vi "QueryServer_SetAnalogInputData.vi"(6 "error in (no error)":errorcluster, 8 "AnalogInputData":T1, 9 "gRPCid":T2) -> (0 "error out":errorcluster, 3 "gRPCid out":T2)   [LabVIEW 2019, in "labview-grpc-query-server.lvlib"]
uses:
  labview-grpc-query-server.lvlib
  VIs/grpcId.ctl
  QueryServer_AnalogInputData.ctl
  d149c175-cf88-4dc1-b2b5-9725cea78de2.vi
  VIs/gprc-support.lvlib
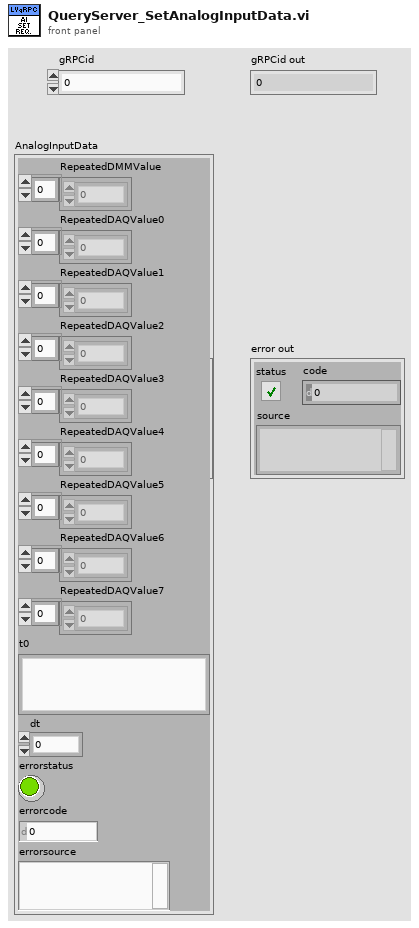
[diagram p1: front panel]
types:
  T1 = typedef "labview-grpc-query-server.lvlib/QueryServer_AnalogInputData.ctl" = cluster{"RepeatedDMMValue":sgl[], "RepeatedDAQValue0":sgl[], "RepeatedDAQValue1":sgl[], "RepeatedDAQValue2":sgl[], "RepeatedDAQValue3":sgl[], "RepeatedDAQValue4":sgl[], "RepeatedDAQValue5":sgl[], "RepeatedDAQValue6":sgl[], "RepeatedDAQValue7":sgl[], "t0":string, "dt":sgl, "errorstatus":bool, "errorcode":i32, "errorsource":string}
  T2 = typedef "gprc-support.lvlib/grpcId.ctl" = u64
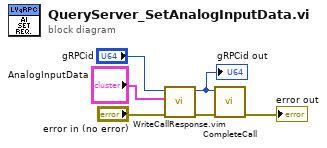
[diagram p0: block diagram]
diagram:
  n1 = call "WriteCallResponse.vim"("error in (no error)"="error in (no error)", "Response Data"="AnalogInputData", "gRPCid in"="gRPCid") -> ("error out"=w5:errorcluster, "gRPCid"=w3:T2)  [unwired: 7 in]
  "gRPCid out" <- w3
  n2 = call "CompleteCall.vi"("gRPCid"=w3, "error in (no error)"=w5) -> ("error out"=→"error out":errorcluster)  [unwired: 8 in]
